vi "ORP_所有参数读取.vi"(8 "error in (no error)":errorcluster caption="错误输入（无错误）", 11 "MB session in":refnum<class "MB_Master.lvclass">) -> (0 "error out":errorcluster caption="错误输出", 2 "输出值":T1 {"电极型号标志" items=["NULL", "pH", "Cond", "DO", "Turb", "ORP"]; "电极状态标志" items=["OK"]}, 3 "MB session out":refnum<class "MB_Master.lvclass">)   [LabVIEW 2016, in "斯坦道多参数.lvlib"]
uses:
  <vilib>/Plasmionique/MB Master/MB_Master/MB_Master.lvclass
  <vilib>/Plasmionique/MB Master/MB Master.lvlib
  <vilib>/ptbypt/NI_PtbyPt.lvlib
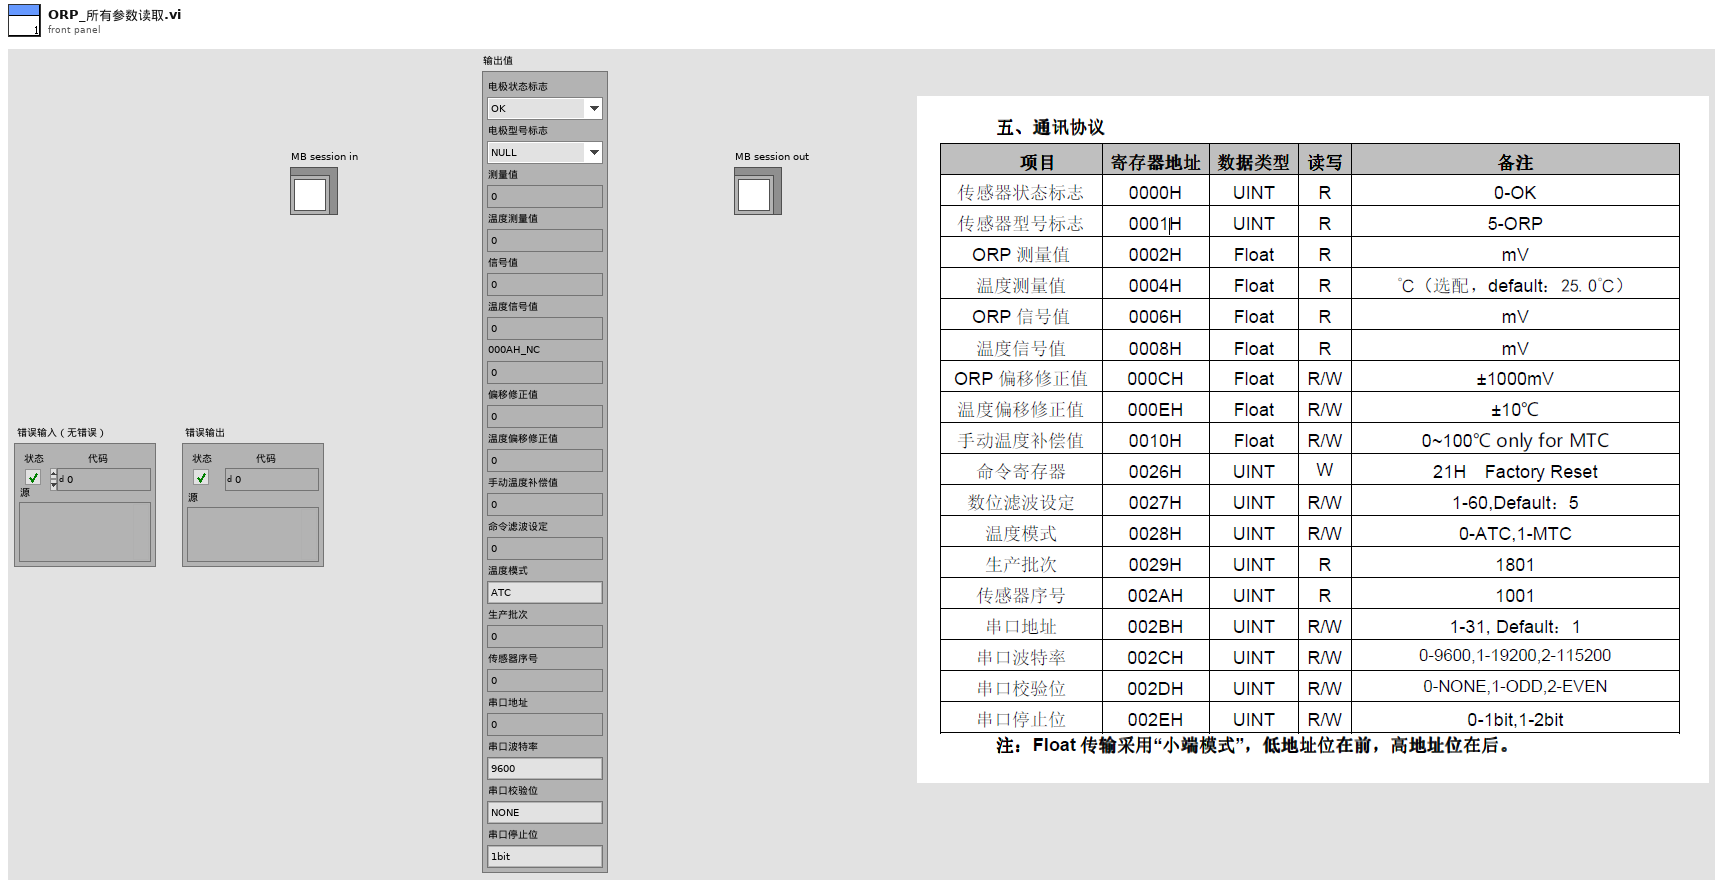
[diagram p1: front panel]
types:
  T1 = cluster{"电极状态标志":u16, "电极型号标志":u16, "测量值":sgl, "温度测量值":sgl, "信号值":sgl, "温度信号值":sgl, "000AH_NC":sgl, "偏移修正值":sgl, "温度偏移修正值":sgl, "手动温度补偿值":sgl, "命令滤波设定":u16, "温度模式":enum16{"ATC", "MTC"}, "生产批次":u16, "传感器序号":u16, "串口地址":u16, "串口波特率":enum16{"9600", "19200", "115200"}, "串口校验位":enum16{"NONE", "ODD", "EVEN"}, "串口停止位":enum16{"1bit", "2bit"}}
  T2 = cluster{u16, u16, "Filtered x":dbl, "数值":sgl, "数值":sgl, "数值":sgl, "数值":sgl, "数值":sgl, "数值":sgl, "数值":sgl, u16, u16, u16, u16, u16, u16, u16, u16}
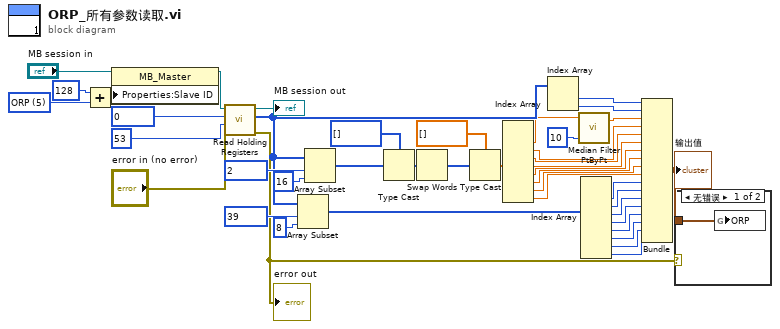
[diagram p0: block diagram]
diagram:
  w43 = u16 5 items=["NULL", "pH", "Cond", "DO", "Turb", "ORP"] ("数值")
  n1 = Add(x=u16 128, y=w43) -> (x+y=w42:u16)
  n2 = property class="MB_Master"(reference="MB session in", "Properties:Slave ID"=w42) -> (reference out=w12:refnum<class "MB_Master.lvclass">)  [unwired: 1 in, 1 out]
  n3 = call <vilib>:"Read Holding Registers.vi"("error in (no error)"="error in (no error)", "quantity"=u16 53, "starting address"=u16 0, "MB session in"=w12) -> ("error out"=w8:errorcluster, "Registers"=w14:u16[], "MB session out"=→"MB session out":refnum<class "MB_Master.lvclass">)  [unwired: 5 in]
  "error out" <- w8
  n4 = Array Subset(array=w14, index=u16 39 ("starting address"), length=8 ("长度")) -> (w23:u16[])
  n5 = Array Subset(array=w14, index=u16 2 ("starting address"), length=16 ("长度")) -> (w31:u16[])
  n6 = Type Cast(type=u32[] [] ("数组 2"), x=w31) -> (*(type *) &x=w33:u32[])
  n7 = Swap Words(1:w33) -> (0:w35:u32[])
  n8 = Type Cast(type=sgl[] [] ("数组 2"), x=w35) -> (*(type *) &x=w30:sgl[])
  n9 = Index Array(array=w30) -> (element #1=w2:sgl, element #2=w29:sgl, element #3=w28:sgl, element #4=w27:sgl, element #5=w11:sgl, element #6=w10:sgl, element #7=w9:sgl, element #8=w5:sgl)  [unwired: 8 in]
  n10 = Index Array(array=w14) -> (element #1=w38:u16, element #2=w37:u16)  [unwired: 2 in]
  n11 = call <vilib>:"Median Filter PtByPt.vi"("rank"=10, "x"=w2) -> ("Filtered x"=w1:dbl)  [unwired: 2 in, 1 out]
  n12 = Index Array(array=w23) -> (element #1=w22:u16, element #2=w21:u16, element #3=w20:u16, element #4=w19:u16, element #5=w18:u16, element #6=w17:u16, element #7=w16:u16, element #8=w15:u16)  [unwired: 8 in]
  n13 = Bundle(w38, w37, "Filtered x"=w1, "数值"=w29, "数值"=w28, "数值"=w27, "数值"=w11, "数值"=w10, "数值"=w9, "数值"=w5, w22, w21, w20, w19, w18, w17, w16, w15) -> (w4:T2)  [unwired: 1 in]
  "输出值" <- w4
  n14 = case shown="无错误" w8 {
    tunnel: w4 -> [w44 _]
    frame No Error {
      n15 = global write "国弘过程全局变量.vi" "ORP"(w44) -> ()
    }
    frame Error {
    }
  }
